vi "Global Stato alimentatori.vi"() -> ()   [LabVIEW 2016]
panel:
  out "Stato alimentatori":T1(array[cluster])
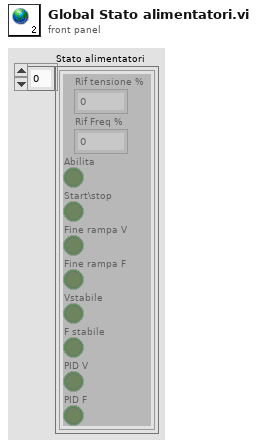
[diagram p1: front panel]
types:
  T1 = cluster{"Rif tensione %":dbl, "Rif Freq %":dbl, "Abilita":bool, "Start\\stop":bool, "Fine rampa V":bool, "Fine rampa F":bool, "Vstabile":bool, "F stabile":bool, "PID V":bool, "PID F":bool}[]
diagram:
